vi "Switch Session Dictionary.vi"(0 "Logical Name":string, 5 "Action":T1, 9 "Ivi Switch Session In":refnum<k15>) -> (4 "Ivi Switch Session Out":refnum<k15>, 6 "Switch session not found / already included":bool, 10 "All Ivi Switch Sessions Out":refnum<k15>[](array[refnum]))   [LabVIEW 2023, in "RFFixtureCharact.RFPM.lvlib" / "RF Subsystem Session Provider.lvclass"]
uses:
  RF Subsystem Session Provider.lvclass
  Common/Data Cache/Type Definitions/Dictionary Operation.ctl
  Common/RFCalAndFixtureCharact.Common.lvlib
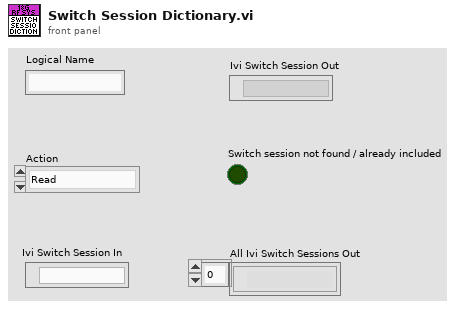
[diagram p1: front panel]
types:
  T1 = typedef "RFCalAndFixtureCharact.Common.lvlib/Dictionary Operation.ctl" = enum16{"Read", "Insert", "Remove", "Clear", "Get All", "Update"}
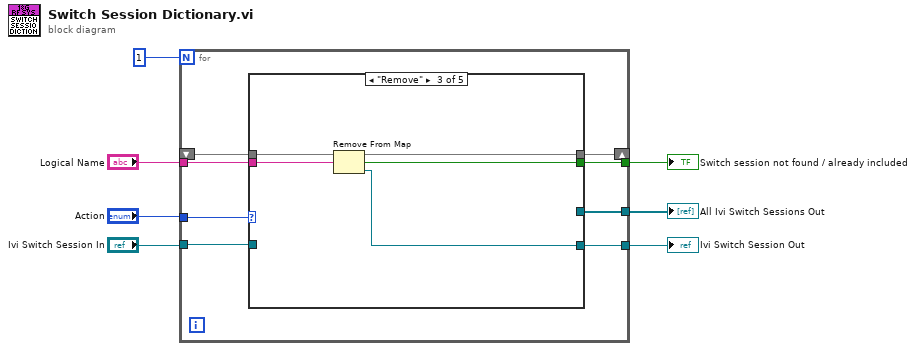
[diagram p0: block diagram]
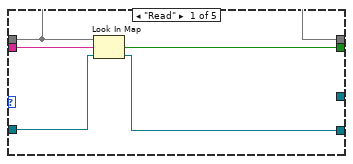
[diagram p2: hidden frame]
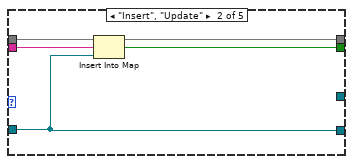
[diagram p3: hidden frame]
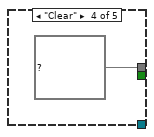
[diagram p4: hidden frame]
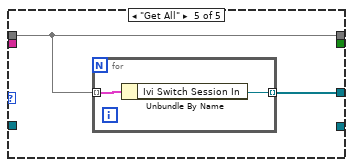
[diagram p5: hidden frame]
diagram:
  n1 = for {
    N: 1 -> [_]
    tunnel: "Action" -> [w15]
    tunnel: "Logical Name" -> [w14]
    tunnel: [w13] -> w6
    tunnel: [w12] -> w1
    shift-right: [w10] -> _
    shift-left: _ -> [w11]
    tunnel: "Ivi Switch Session In" -> [w9]
    tunnel: [w8] -> w4
    n2 = case shown="\"Remove\"" w15 {
      tunnel: w14 -> [w20 w25 w28 _ _]
      tunnel: w11 -> [w18 w24 w29 _ w33]
      tunnel: [w19 w23 w30 _ _] -> w13
      tunnel: [w16 w21 w27 _ _] -> w12
      tunnel: [w18 w22 w26 map{string, refnum<k15>} {} ("map") w33] -> w10
      tunnel: w9 -> [w17 w21 _ _ _]
      tunnel: [_ _ _ _ w32] -> w8
      frame "Read" {
        n3 = Look In Map(map=w18, key=w20, default value=w17) -> (key not found?=w19:bool, value=w16:refnum<k15>)
      }
      frame "Insert", "Update" {
        n4 = Insert Into Map(map in=w24, key=w25, value=w21) -> (map out=w22:map{string, refnum<k15>}, key already included?=w23:bool)  [unwired: 1 out]
      }
      frame "Remove" {
        n5 = Remove From Map(10:w28, 11:w29) -> (1:w27:refnum<k15>, 2:w30:bool, 3:w26:map{string, refnum<k15>})
      }
      frame "Clear" {
      }
      frame "Get All" {
        n6 = for {
          tunnel: [w34] -> w32 mode=indexing
          tunnel: w33 -> [w35] mode=indexing
          n7 = Unbundle By Name(w35) -> ("Ivi Switch Session In"=w34:refnum<k15>)
        }
      }
    }
  }
  "Switch session not found / already included" <- w6
  "All Ivi Switch Sessions Out" <- w4
  "Ivi Switch Session Out" <- w1
